vi "TCP设备参数设置.vi"(8 "布尔文本.文本":string, 9 "section (optional)":string, 10 "监测项描述":string) -> (2 "布尔":bool=TRUE, 3 "输出簇":T2)   [LabVIEW 2016, in "环境动力监测库.lvlib"]
uses:
  <vilib>/Utility/miscctls.llb/LVPointTypeDef.ctl
  <vilib>/Utility/config.llb/NI_LVConfig.lvlib
panel:
  in  "Port:":string
  in  "data bits":u64=8 caption="数据比特" min=5 max=8 step=1
  in  "波特率":u64=19200
  in  "停止位":u16(ring)=10 items=["1.0"=10, "1.5"=15, "2.0"=20]
  in  "奇偶校验":u16(ring) items=["None", "Odd", "Even", "Mark", "Space"]
  in  "传感器型号:":T1(ring)
  in  "输入簇":T2
  in  "站号":u64
  in  "返回":bool
  in  "增加":bool
  in  "IP address:":string
  in  "监测项描述:":string
  # "基本设置"
  # "如:红外XX"
  # "传感器选择"
  # "地址选择"
  # "站号配置"
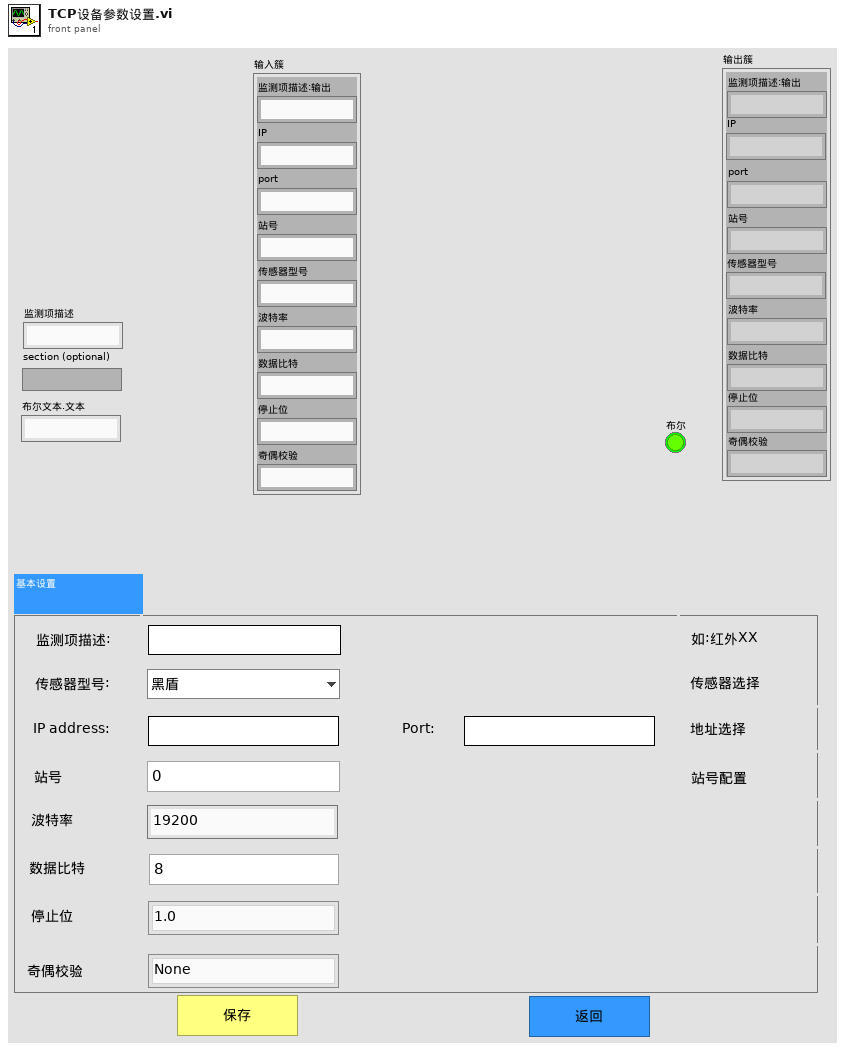
[diagram p1: front panel]
types:
  T1 = enum16{"黑盾", "英维克", "梦幻城堡C6~20KS", "梦幻城堡C1K(S)~C3K(S)"}
  T2 = cluster{"监测项描述:输出":string, "IP":string, "port":string, "站号":string, "传感器型号":string, "波特率":string, "数据比特":string, "停止位":string, "奇偶校验":string}
  T3 = typedef "LVPointTypeDef.ctl" = cluster{"Horizontal":i16, "Vertical":i16}
  T4 = typedef "NI_LVConfig.lvlib/Config Data RefNum.ctl" = refnum<k1>
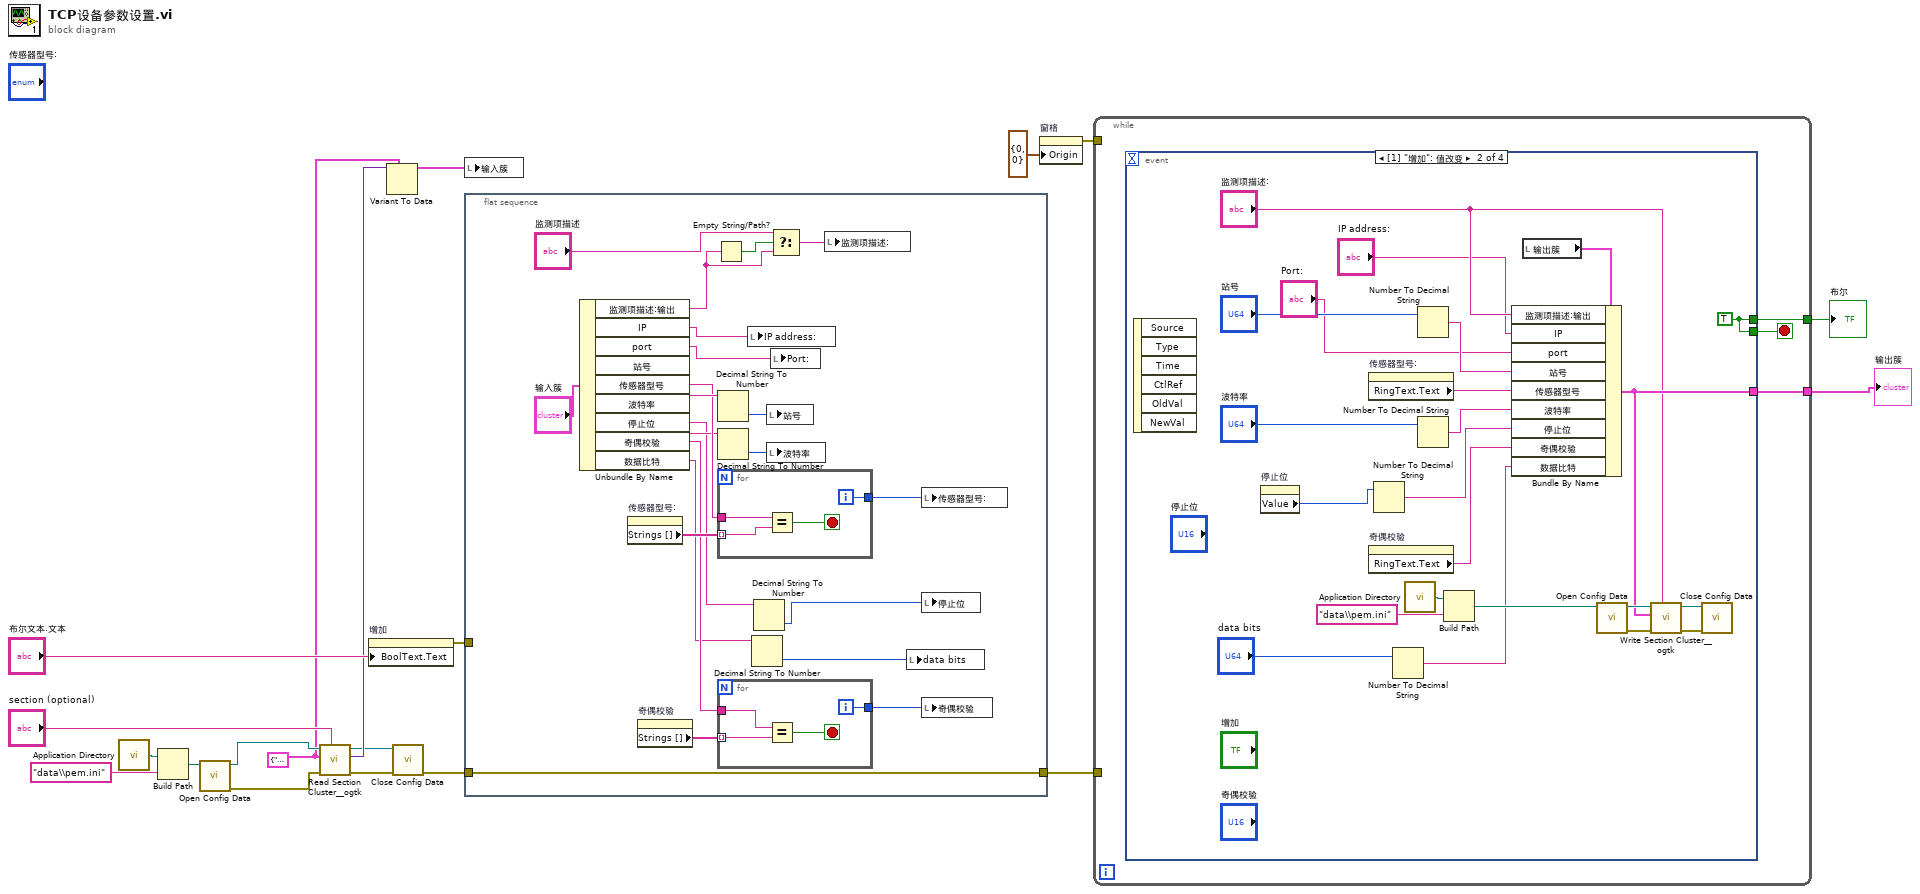
[diagram p0: block diagram]
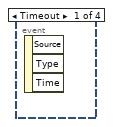
[diagram p2: hidden frame]
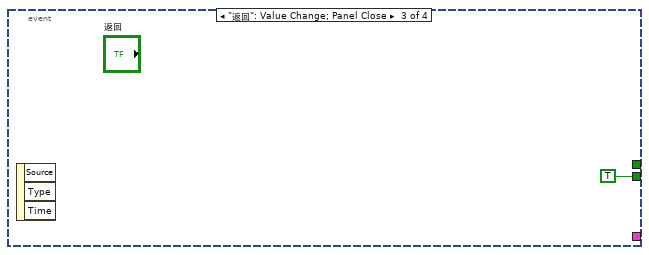
[diagram p3: hidden frame]
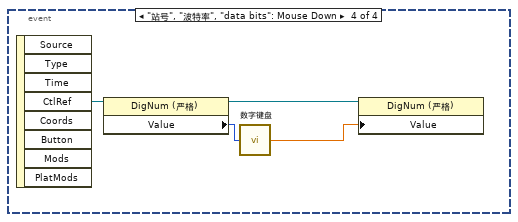
[diagram p4: hidden frame]
diagram:
  w1 = T2 {"监测项描述:输出"="", "IP"="", "port"="", "站号"="", "传感器型号"="", "波特率"="", "数据比特"="", "停止位"="", "奇偶校验"=""} ("数据")
  n1 = call <vilib>:"Application Directory.vi"() -> ("Application Directory"=w12:path)
  n2 = Build Path(base path=w12, name or relative path="data\\pem.ini" ("名称或相对路径")) -> (appended path=w13:path)
  n3 = call <vilib>:"Open Config Data.vi"("configuration file path"=w13) -> ("error out"=w14:errorcluster, "refnum"=w15:T4)  [unwired: 8 in, 1 out]
  n4 = call <userlib>:"Read Section Cluster__ogtk.vi"("section (optional)"="section (optional)", "error in (no error)"=w14, "Section Formatted Cluster Type"=w1, "refnum"=w15) -> ("error out"=w6:errorcluster, "Section Formatted Cluster"=w9:variant, "dup refnum"=w7:T4)  [unwired: 3 in, 2 out]
  n5 = property on="增加" class="Bool"("BoolText.Text"="布尔文本.文本") -> (error out=w5:errorcluster)  [unwired: 2 in, 1 out]
  n6 = Variant To Data(type=w1, Variant=w9) -> (data=w8:T2)  [unwired: 1 in, 1 out]
  n7 = call <vilib>:"Close Config Data.vi"("error in (no error)"=w6, "refnum"=w7) -> ("error out"=w4:errorcluster)  [unwired: 8 in, 1 out]
  n8 = local write "输入簇"(w8) -> ()
  n9 = flat-sequence {
    tunnel: w5 -> [_]
    tunnel: w4 -> [w39]
    tunnel: [w39] -> w3
    frame #0 {
      n10 = Unbundle By Name("输入簇") -> ("监测项描述:输出"=w22:string, "IP"=w21:string, "port"=w20:string, "站号"=w40:string, "传感器型号"=w33:string, "波特率"=w30:string, "停止位"=w26:string, "奇偶校验"=w27:string, "数据比特"=w24:string)
      n11 = property on="传感器型号:" class="Enum (严格)"() -> ("Strings []"=w34:string[])  [unwired: 2 in, 2 out]
      n12 = property on="奇偶校验" class="Ring (严格)"() -> ("Strings []"=w28:string[])  [unwired: 2 in, 2 out]
      n13 = Empty String/Path?(string/path=w22) -> (empty?=w38:bool)
      n14 = Decimal String To Number(string=w40) -> (number=w35:i32)  [unwired: 2 in, 1 out]
      n15 = Decimal String To Number(string=w30) -> (number=w31:i32)  [unwired: 2 in, 1 out]
      n16 = for {
        tunnel: w33 -> [w49]
        tunnel: [w47] -> w32
        tunnel: w34 -> [w46] mode=indexing
        i -> [w47]
        stop <- w48 stop-if-true
        n17 = Equal?(x=w49, y=w46) -> (x = y?=w48:bool)
      }
      n18 = for {
        tunnel: w27 -> [w45]
        tunnel: [w43] -> w29
        tunnel: w28 -> [w42] mode=indexing
        i -> [w43]
        stop <- w44 stop-if-true
        n19 = Equal?(x=w45, y=w42) -> (x = y?=w44:bool)
      }
      n20 = local write "IP address:"(w21) -> ()
      n21 = Decimal String To Number(string=w24) -> (number=w23:i32)  [unwired: 2 in, 1 out]
      n22 = Decimal String To Number(string=w26) -> (number=w25:i32)  [unwired: 2 in, 1 out]
      n23 = local write "站号"(w35) -> ()
      n24 = local write "波特率"(w31) -> ()
      n25 = Select(t="监测项描述", s=w38, f=w22) -> (s? t:f=w36:string)
      n26 = local write "Port:"(w20) -> ()
      n27 = local write "监测项描述:"(w36) -> ()
      n28 = local write "data bits"(w23) -> ()
      n29 = local write "传感器型号:"(w32) -> ()
      n30 = local write "停止位"(w25) -> ()
      n31 = local write "奇偶校验"(w29) -> ()
    }
  }
  n32 = property on="窗格" class="Pane"("Origin"=T3 {"Horizontal"=0, "Vertical"=0} ("原点")) -> (error out=w19:errorcluster)  [unwired: 2 in, 1 out]
  n33 = while {
    tunnel: w19 -> [_]
    tunnel: [w52] -> w2
    tunnel: [w50] -> w17
    tunnel: w3 -> [_]
    stop <- w51 stop-if-true
    n34 = event shown="[1] \"增加\": 值改变" {
      selector: _ -> [_ _ _ _]
      dyn-events: _ -> [_ _ _ _]
      timeout: _ -> [_ _ _ _]
      tunnel: [_ w68 _ _] -> w52
      tunnel: [_ w67 TRUE _] -> w51
      tunnel: [_ w67 _ _] -> w50
      event Timeout {
        n35 = event-data() -> ()  [unwired: 1 in, 3 out]
      }
      event "增加": Value Change {
        w67 = TRUE
        n36 = event-data() -> ()  [unwired: 1 in, 6 out]
        n37 = property on="停止位" class="Ring (严格)"() -> ("Value"=w60:u16)  [unwired: 2 in, 2 out]
        n38 = property on="传感器型号:" class="Enum (严格)"() -> ("RingText.Text"=w64:string)  [unwired: 2 in, 2 out]
        n39 = property on="奇偶校验" class="Ring (严格)"() -> ("RingText.Text"=w61:string)  [unwired: 2 in, 2 out]
        n40 = Number To Decimal String(number=w60) -> (decimal integer string=w59:string)  [unwired: 1 in]
        n41 = Number To Decimal String(number="data bits") -> (decimal integer string=w58:string)  [unwired: 1 in]
        n42 = call <vilib>:"Application Directory.vi"() -> ("Application Directory"=w72:path)
        n43 = Number To Decimal String(number="站号") -> (decimal integer string=w66:string)  [unwired: 1 in]
        n44 = Number To Decimal String(number="波特率") -> (decimal integer string=w62:string)  [unwired: 1 in]
        n45 = Build Path(base path=w72, name or relative path="data\\pem.ini" ("名称或相对路径")) -> (appended path=w73:path)
        n46 = local read "输出簇"() -> (w53:T2)
        n47 = Bundle By Name(cluster=w53, "监测项描述:输出"="监测项描述:", "IP"="IP address:", "port"="Port:", "站号"=w66, "传感器型号"=w64, "波特率"=w62, "停止位"=w59, "奇偶校验"=w61, "数据比特"=w58) -> (w68:T2)
        n48 = call <vilib>:"Open Config Data.vi"("configuration file path"=w73) -> ("error out"=w74:errorcluster, "refnum"=w75:T4)  [unwired: 8 in, 1 out]
        n49 = call <userlib>:"Write Section Cluster__ogtk.vi"("section (optional)"="监测项描述:", "error in (no error)"=w74, "Section Formatted Cluster"=w68, "refnum"=w75) -> ("error out"=w69:errorcluster, "dup refnum"=w70:T4)  [unwired: 6 in]
        n50 = call <vilib>:"Close Config Data.vi"("error in (no error)"=w69, "refnum"=w70) -> ()  [unwired: 8 in, 2 out]
      }
      event "返回": Value Change; Panel Close {
        n51 = event-data() -> ()  [unwired: 1 in, 3 out]
      }
      event "站号", "波特率", "data bits": Mouse Down {
        n52 = event-data() -> ("CtlRef"=w80:refnum<vi>)  [unwired: 1 in, 7 out]
        n53 = property class="DigNum (严格)"(reference=w80) -> (reference out=w78:refnum<vi>, "Value"=w79:u64)  [unwired: 1 in, 1 out]
        n54 = call "数字键盘.vi"("OldNumber"=w79) -> ("NewNumber"=w77:sgl)
        n55 = property class="DigNum (严格)"(reference=w78, "Value"=w77) -> ()  [unwired: 1 in, 2 out]
      }
    }
  }
  "输出簇" <- w2
  "布尔" <- w17
